vi "CSM - Wait for All Modules to be Alive.vi"(6 "Wait (5000 ms)":u32=5000, 8 "Error In":errorcluster caption="error in (no error)", 11 "CSM Names":string[](array[string])) -> (0 "error out":errorcluster, 1 "Waited (ms)":u32, 2 "CSMs Left":string[](array[string]))   [LabVIEW 2017, in "Communicable State Machine.lvlib"]
doc: "Waits for a group of CSM modules to all come online within a specified timeout period, and returns the wait time. This VI returns an error and the names of modules that did not come online if the timeout is exceeded. Internally, this VI periodically checks if all modules are online using the CSM - List Module VI at 5 ms intervals.\n\n-- <b>Controls</b> --\n- <b>CSM Names</b>: CSM module names.\n- <b>Timeout (5000ms)</b>: Timeout duration for waiting. The default is 5000 ms.\n\n-- <b>Indicators</b> --\n- <b>CSMs Left</b>: CSM modules that have not come online after the timeout.\n- <b>Waited (ms)</b>: Time elapsed while waiting."
uses:
  Communicable State Machine.lvlib
  _Support/Typedef/_CSM_List Module Scope.ctl
  _Shared/CSM Shared.lvlib
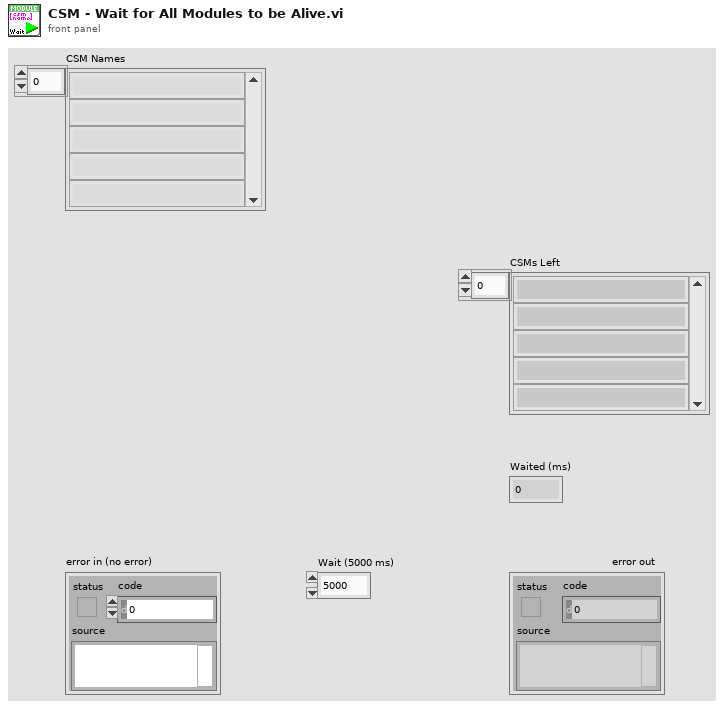
[diagram p1: front panel]
types:
  T1 = typedef "Communicable State Machine.lvlib/_CSM_List Module Scope.ctl" = enum16{"Normal", "System Only", "All"}
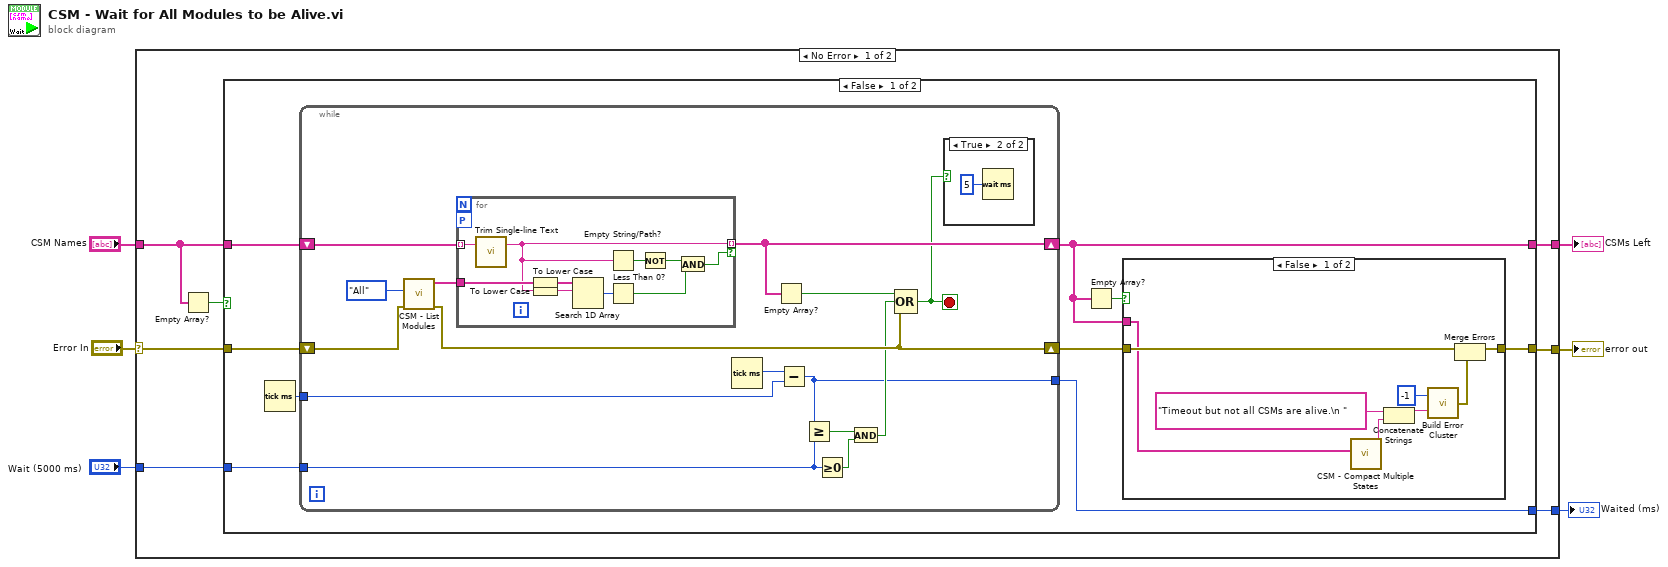
[diagram p0: block diagram]
diagram:
  n1 = case shown="No Error" "Error In" {
    selector: "Error In" -> [w13 w61]
    tunnel: [w11 w61] -> w5
    tunnel: "CSM Names" -> [w8 w60]
    tunnel: [w10 w60] -> w3
    tunnel: "Wait (5000 ms)" -> [w12 _]
    tunnel: [w7 _] -> w1
    frame No Error {
      n2 = Empty Array?(array=w8) -> (empty?=w9:bool)
      n3 = case shown="False" w9 {
        tunnel: w8 -> [w22 w59]
        tunnel: w13 -> [w21 w58]
        tunnel: w12 -> [w19 _]
        tunnel: [w17 w58] -> w11
        tunnel: [w15 w59] -> w10
        tunnel: [w14 _] -> w7
        frame False {
          n4 = Tick Count (ms)() -> (millisecond timer value=w20:u32)
          n5 = while {
            shift-right: [w44] -> w15
            shift-left: w22 -> [w46]
            shift-right: [w41] -> w16
            shift-left: w21 -> [w43]
            tunnel: w20 -> [w40]
            tunnel: w19 -> [w38]
            tunnel: [w33] -> w14
            stop <- w39 stop-if-true
            n6 = call "CSM - List Modules.vi"("Error In"=w43, "Scope (Normal)"=_CSM_List_Module_Scope."All" ("Mode")) -> ("error out"=w41:errorcluster, "Module Names"=w45:string[])  [unwired: 8 in]
            n7 = for {
              tunnel: w46 -> [w53] mode=indexing
              tunnel: w45 -> [w57]
              tunnel: [w49] -> w44 mode=indexing if=w51
              workers-P: _ -> [_]
              n8 = call "Trim Single-line Text.vi"("single-line text"=w53) -> ("trimed text"=w49:string)  [unwired: 2 in]
              n9 = To Lower Case(string=w57) -> (all lower case string=w55:string[])
              n10 = To Lower Case(string=w49) -> (all lower case string=w54:string)
              n11 = Search 1D Array(1D array=w55, element=w54) -> (index of element=w56:i32)  [unwired: 1 in]
              n12 = Empty String/Path?(string/path=w49) -> (empty?=w50:bool)
              n13 = Less Than 0?(x=w56) -> (x < 0?=w52:bool)
              n14 = Not(x=w50) -> (.not. x?=w48:bool)
              n15 = And(x=w48, y=w52) -> (x .and. y?=w51:bool)
            }
            n16 = Tick Count (ms)() -> (millisecond timer value=w37:u32)
            n17 = Empty Array?(array=w44) -> (empty?=w42:bool)
            n18 = Subtract(x=w37, y=w40) -> (x-y=w33:u32)
            n19 = Greater Or Equal?(x=w33, y=w38) -> (x >= y?=w35:bool)
            n20 = Greater Or Equal To 0?(x=w38) -> (x >= 0?=w34:bool)
            n21 = And(x=w35, y=w34) -> (x .and. y?=w36:bool)
            n22 = Compound Arithmetic op=OR(w42, w36, w41) -> (w39:bool)
            n23 = case shown="True" w39 {
              frame False {
              }
              frame True {
                n24 = Wait (ms)(milliseconds to wait=u32 5) -> ()  [unwired: 1 out]
              }
            }
          }
          n25 = Empty Array?(array=w15) -> (empty?=w18:bool)
          n26 = case shown="False" w18 {
            tunnel: [w29 w31] -> w17
            tunnel: w16 -> [w30 w31]
            tunnel: w15 -> [w24 _]
            frame False {
              n27 = call "CSM - Compact Multiple States.vi"("Multiple States"=w24) -> ("States"=w23:string)  [unwired: 9 in]
              n28 = Concatenate Strings("Timeout but not all CSMs are alive.\n " ("String to Prepend to source (\"\")"), w23) -> (w25:string)
              n29 = call "Build Error Cluster.vi"("String to Prepend to Source (\"\")"=w25, "Code"=-1 ("code")) -> ("error out"=w28:errorcluster)
              n30 = Merge Errors(w30, w28) -> (w29:errorcluster)
            }
            frame True {
            }
          }
        }
        frame True {
        }
      }
    }
    frame Error {
    }
  }
  "error out" <- w5
  "CSMs Left" <- w3
  "Waited (ms)" <- w1
